vi "Gantner_Get Module List.vi"(8 "error in":errorcluster caption="Fehler (Eingang - kein Fehler)") -> (0 "error out":errorcluster caption="error in", 3 "ModuleArray":T1[](array[typedef]))   [LabVIEW 2016]
uses:
  HardWare/Gantner/GantnerDriver/Gantner-Instruments ISMBUS32/ISMBUS_Module.ctl
  HardWare/Gantner/GantnerDriver/Gantner-Instruments ISMBUS32/ISMBUS_Channel.ctl
  ISMBUS32.DLL
panel:
  out "ItemList 2":i32[](array[numeric])
  out "ItemListItemSub1":i32
  out "ItemList":i32[](array[numeric])
  out "ItemCount":i32
  out "StructureID":i32
  out "AddArgument":i32
  out "MaxScanCount":i32
  out "ScanBaudrate":i32
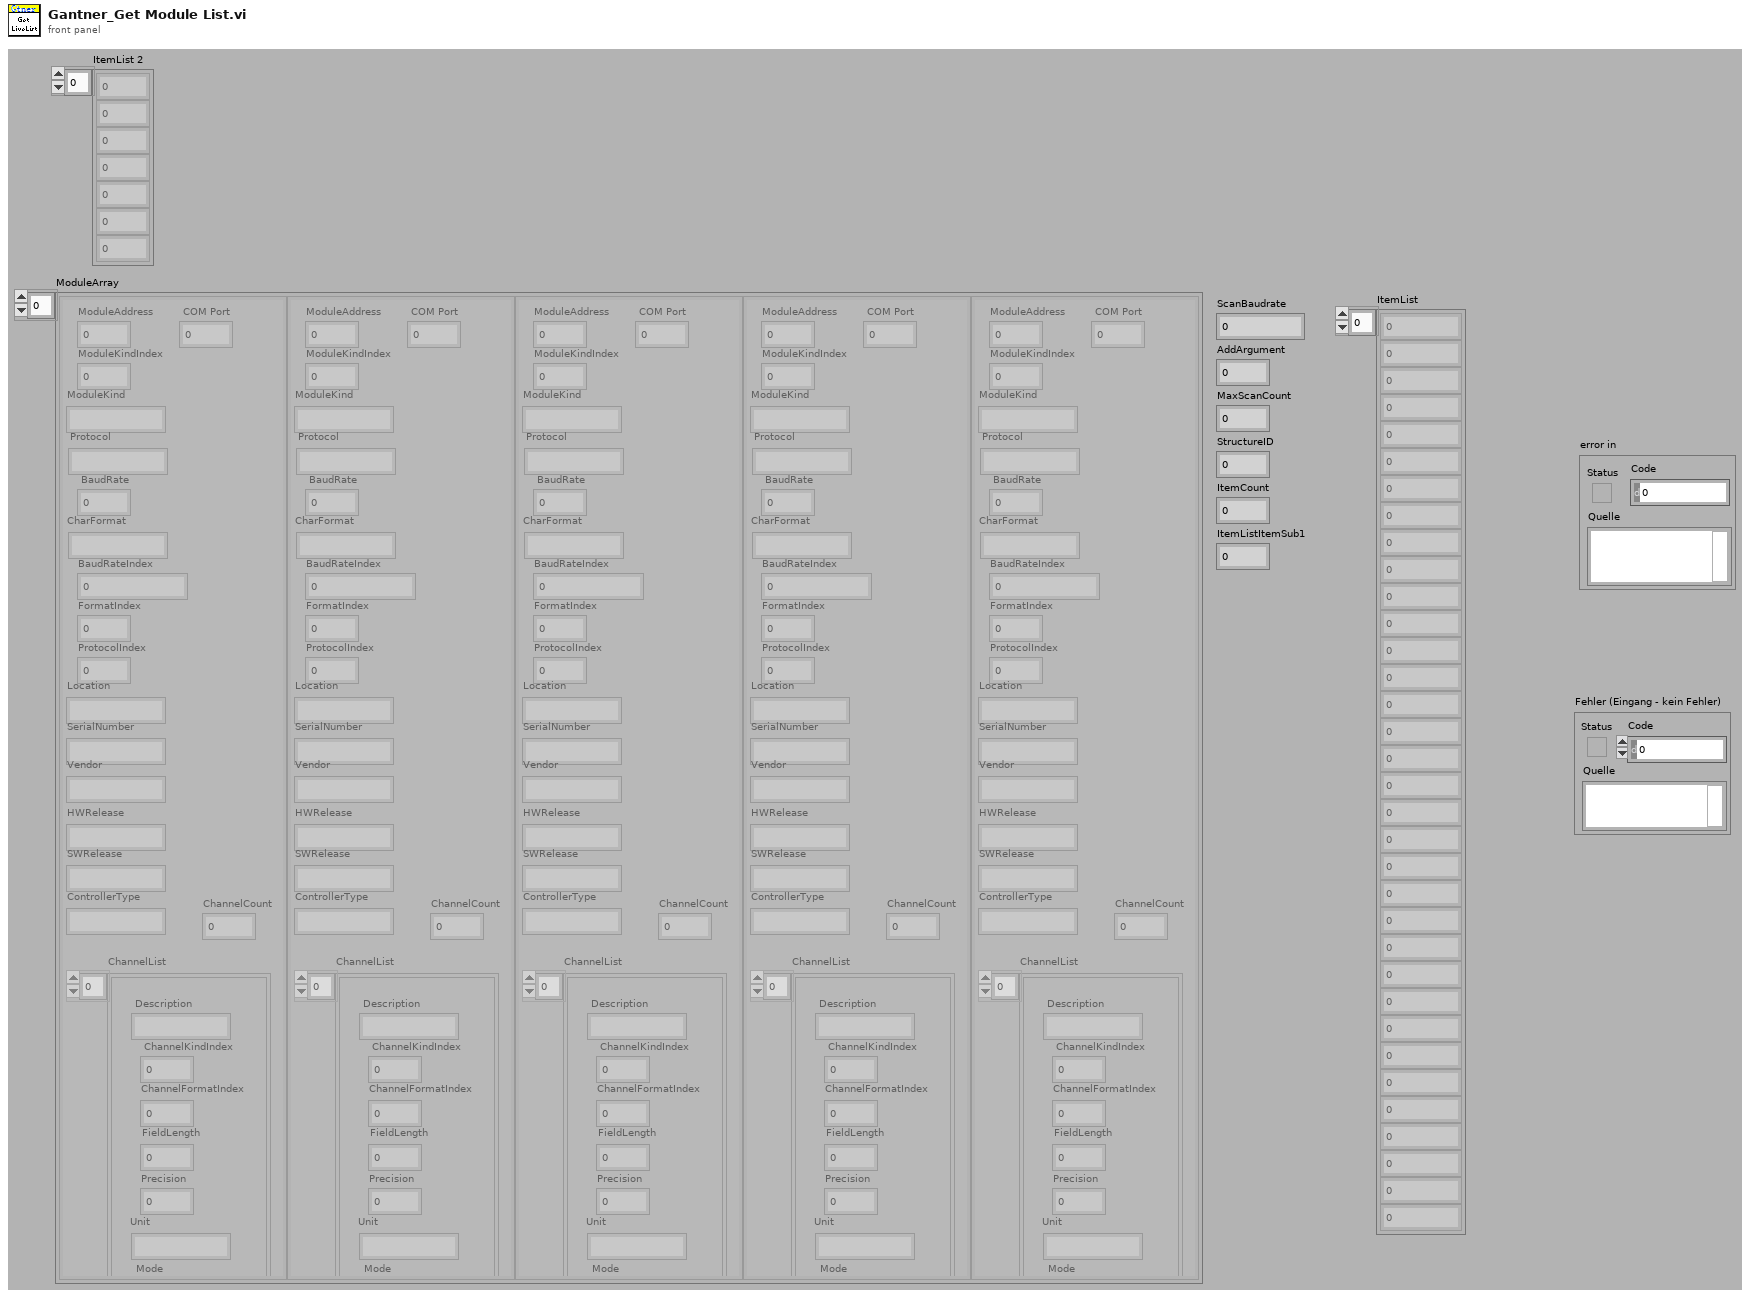
[diagram p1: front panel]
types:
  T1 = typedef "ISMBUS_Module.ctl" = cluster{"ModuleAddress":i32, "ModuleKindIndex":i32, "ModuleKind":string, " Protocol":string, " BaudRate":i32, "CharFormat":string, "BaudRateIndex":i32, "FormatIndex":i32, "ProtocolIndex":i32, "Location":string, "SerialNumber":string, "Vendor":string, "HWRelease":string, "SWRelease":string, "ControllerType":string, "ChannelList":T2[], "ChannelCount":i32, " COM Port":i32}
  T2 = typedef "ISMBUS_Channel.ctl" = cluster{" Description":string, " ChannelKindIndex":i32, "ChannelFormatIndex":i32, " FieldLength":i32, "Precision":i32, "Unit":string, "Mode":i32}
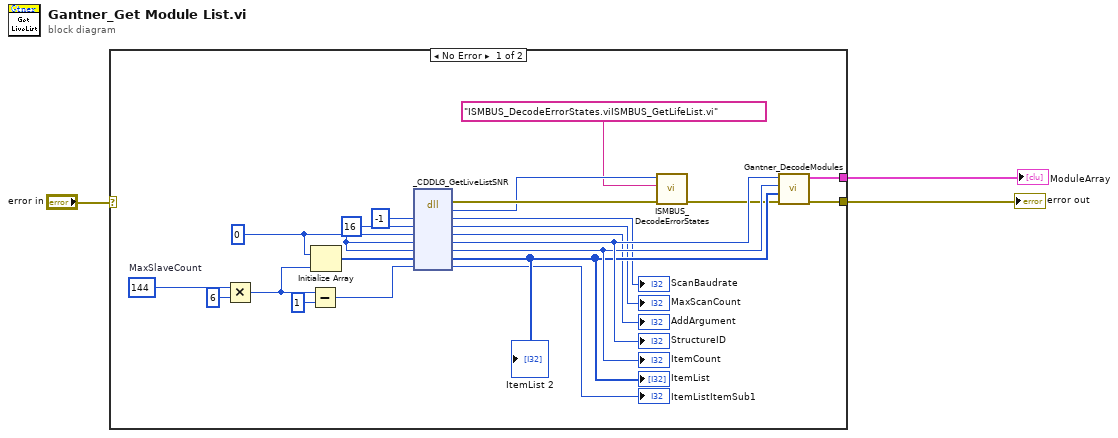
[diagram p0: block diagram]
diagram:
  n1 = case shown="No Error" "error in" {
    selector: "error in" -> [_ w26]
    tunnel: [w16 w26] -> w1
    tunnel: [w11 _] -> w2
    frame No Error {
      w4 = 0 ("AddArgument")
      w22 = 144  # MaxSlaveCount
      n2 = Multiply(x=w22, y=6) -> (x*y=w20:i32)
      n3 = Subtract(x=w20, y=1) -> (x-y=w17:i32)
      n4 = Initialize Array(w4, w20) -> (w18:i32[])
      n5 = dll-call lib="Ismbus32.dll" fn="_CDDLG_GetLiveListSNR"("ScanBaudrate"=-1, "MaxScanCount"=16, "AddArgument"=w4, "StructureID"=w4, "ItemCount"=w4, "ItemList"=w18, "ItemListItemSub1"=w17) -> (error out=w15:errorcluster, "Rückgabetyp"=w14:i32, "ScanBaudrate"=→"ScanBaudrate":i32, "MaxScanCount"=→"MaxScanCount":i32, "AddArgument"=→"AddArgument":i32, "StructureID"=w25:i32, "ItemCount"=w24:i32, "ItemList"=w23:i32[], "ItemListItemSub1"=→"ItemListItemSub1":i32)  [unwired: 3 in, 1 out]
      "StructureID" <- w25
      "ItemCount" <- w24
      "ItemList" <- w23
      "ItemList 2" <- w23
      n6 = call "ISMBUS_DecodeErrorStates.vi"("Fehler (Eingang - kein Fehler)"=w15, "Location"="ISMBUS_DecodeErrorStates.viISMBUS_GetLifeList.vi", "ISMBUS_Error State"=w14) -> ("Fehler (Ausgang)"=w13:errorcluster)  [unwired: 8 out]
      n7 = call "Gantner_DecodeModules.vi"("error in"=w13, "Array"=w23, "ItemsCount"=w24, "Stricture ID"=w25) -> ("error out"=w16:errorcluster, "ModuleArray"=w11:T1[])  [unwired: 6 in]
    }
    frame Error {
    }
  }
  "ModuleArray" <- w2
  "error out" <- w1
